vi "SVA 4MV6 T024 CCE.vi"() -> ()   [LabVIEW 2020]
doc: "Ceballos Conde Emanuelm 4MV6 Sistemas de visión artificial 2022/1\nEste vi realiza el control difuso SIMO del sitema de orientacion de un robot lego untilizando el REPERTORIO DE FUNCIONES DEL TOOL KIT FUZZY LOGIC DE LABVIEW."
uses:
  <vilib>/addons/Fuzzy Logic/TypeDefs/FL Defuzzification.ctl
  <vilib>/addons/Fuzzy Logic/TypeDefs/FL Antecedent Connective.ctl
  <vilib>/addons/Fuzzy Logic/TypeDefs/FL Consequent Implication.ctl
  <vilib>/addons/Fuzzy Logic/TypeDefs/FL Modifier.ctl
  <vilib>/addons/Fuzzy Logic/Membership/FL Create Membership Function (Triangle).vi
  <vilib>/addons/Fuzzy Logic/Membership/FL Create Membership Function (Trapezoid).vi
  <vilib>/addons/Fuzzy Logic/FL Fuzzy Controller (SIMO).vi
  <vilib>/addons/Fuzzy Logic/NI_Fuzzy_Logic_API.lvlib
panel:
  out "output values":dbl[](array[numeric])
  out "distancia":dbl(slide) scale=0.0..100.0
  out "angulo":dbl(knob) scale=-25.0..25.0
  in  "Reset":bool
  out "Motor Izquierda":dbl(slide) scale=-100.0..100.0
  out "Motor Derecha":dbl(slide) scale=-100.0..100.0
  out "Plano de trabajo":picture
  in  "stop":bool
  # "Ceballos Conde Emanuel\n4MV6\nSistemas de visión artificial\n2022/1"
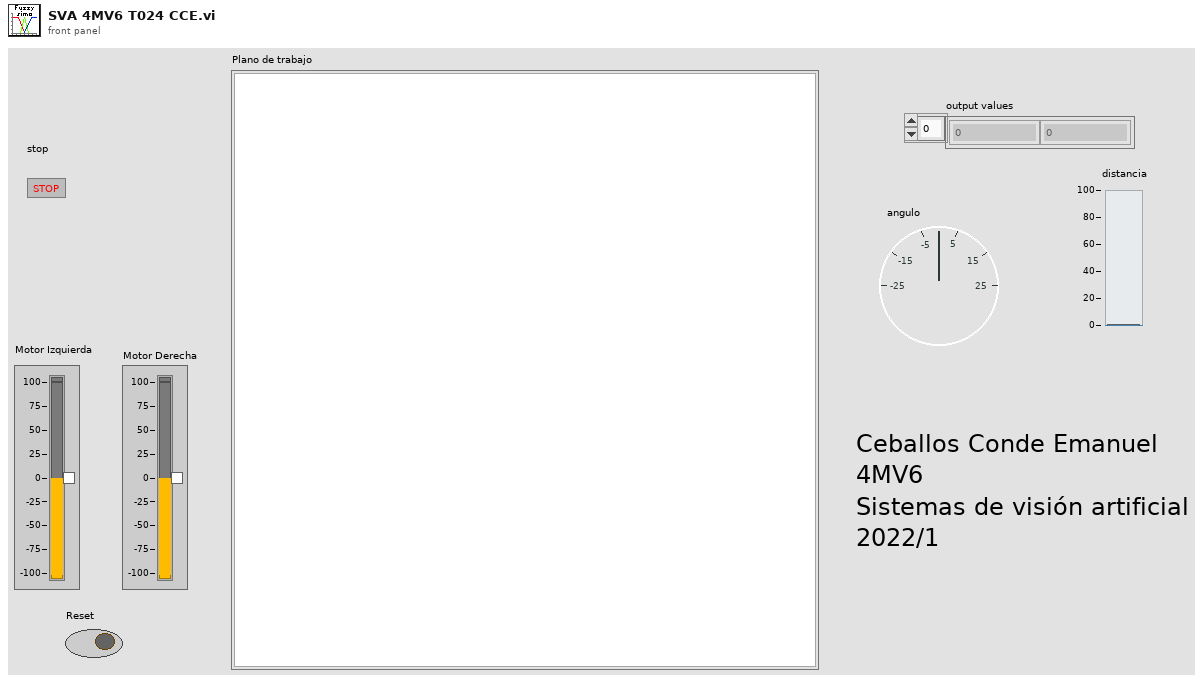
[diagram p1: front panel]
types:
  T1 = typedef "NI_Fuzzy_Logic_API.lvlib/FL Defuzzification.ctl" = u16
  T2 = typedef "NI_Fuzzy_Logic_API.lvlib/FL Membership Function.ctl" = cluster{"name":string, "shape":T3, "points":dbl[], "color":u32, "user-defined shape index":i32}
  T3 = typedef "NI_Fuzzy_Logic_API.lvlib/FL Membership Function Shape.ctl" = u16
  T4 = typedef "NI_Fuzzy_Logic_API.lvlib/FL Variable.ctl" = cluster{"name":string, "range":dbl[], "MFs":T2[]}
  T5 = typedef "NI_Fuzzy_Logic_API.lvlib/FL Modifier.ctl" = u16
  T6 = typedef "NI_Fuzzy_Logic_API.lvlib/FL Consequent Implication.ctl" = u16
  T7 = typedef "NI_Fuzzy_Logic_API.lvlib/FL Antecedent Connective.ctl" = u16
  T8 = typedef "NI_Fuzzy_Logic_API.lvlib/FL Consequent.ctl" = cluster{"Var Index":i32, "MF Index":i32, "Cond":T5}
  T9 = typedef "NI_Fuzzy_Logic_API.lvlib/FL Antecedent.ctl" = cluster{"Var Index":i32, "MF Index":i32, "Cond":T5}
  T10 = typedef "NI_Fuzzy_Logic_API.lvlib/FL Rule.ctl" = cluster{"antecedents":T9[], "antecedent connective":T7, "consequents":T8[], "consequent implication":T6, "degree of support":dbl}
  T11 = typedef "NI_Fuzzy_Logic_API.lvlib/FL System.ctl" = cluster{"input variables":T4[], "output variables":T4[], "rules":T10[], "defuzzification method":T1, "description":string, "user MF interpolating polynomials":T12[]}
  T12 = typedef "NI_Fuzzy_Logic_API.lvlib/FL Interpolating polynomials.ctl" = cluster{"X":dbl[], "Y":dbl[], "Y(x) coeff":dbl[][], "X(y) coeff":dbl[][], "Area(y) coeff":dbl[][], "coa_x(y) coeff":dbl[][]}
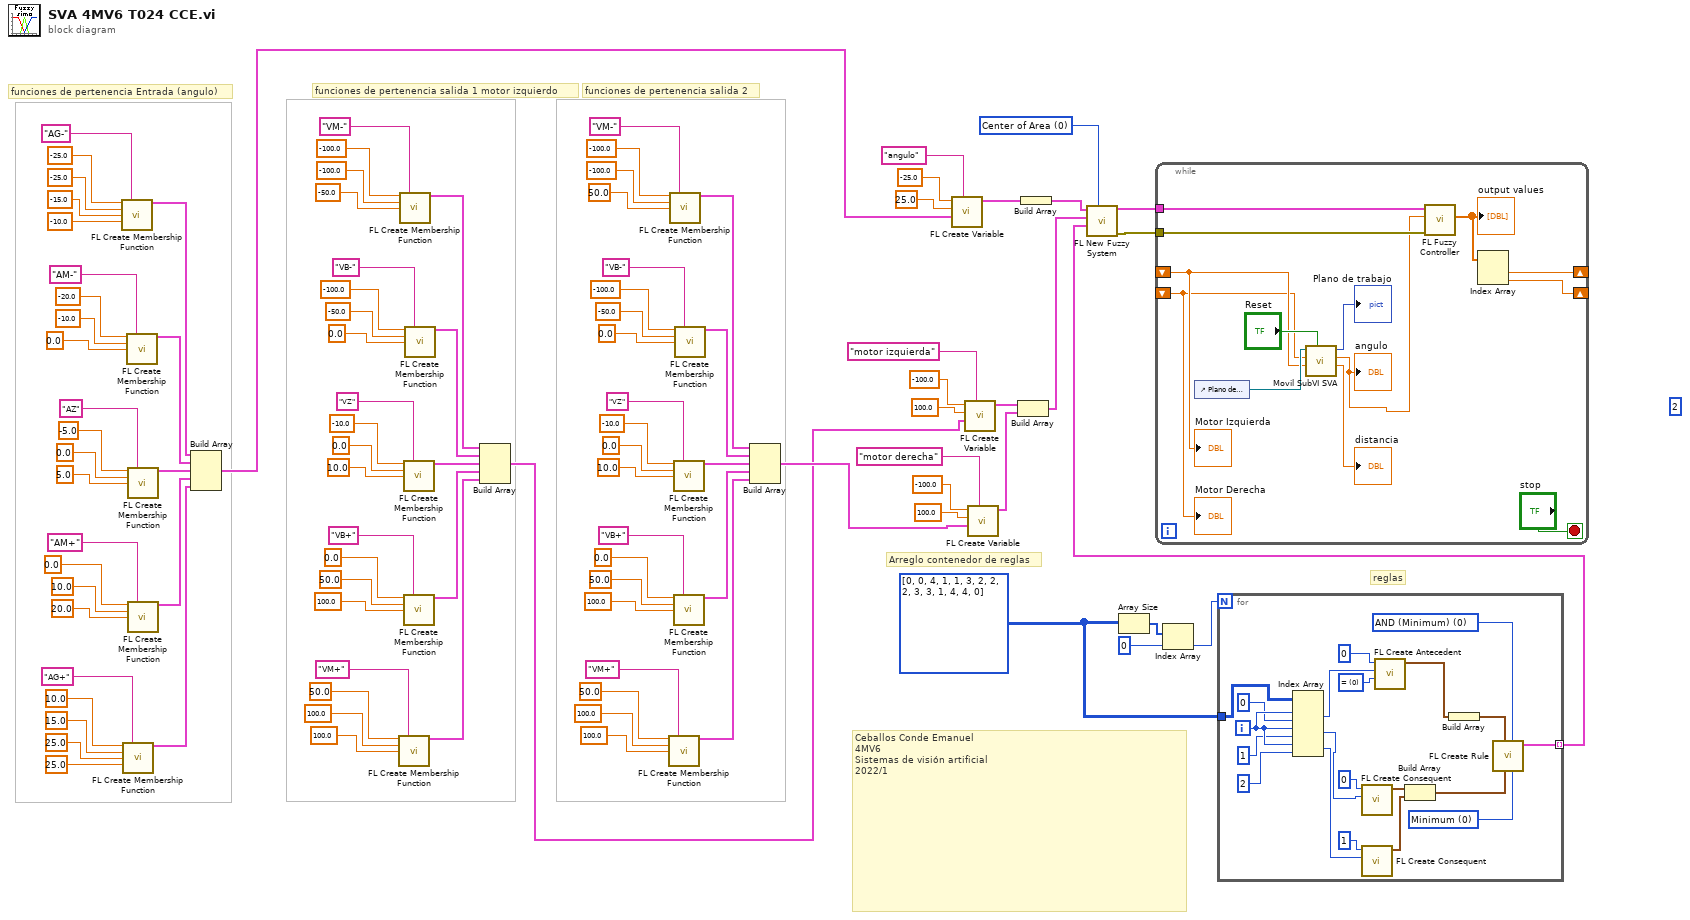
[diagram p0: block diagram]
diagram:
  (unwired) 2
  w4 = i32[][] [[0, 0, 4], [1, 1, 3], [2, 2, 2], [3, 3, 1], [4, 4, 0]]
  w100 = T1 0 items=["Center of Area", "Modified Center of Area", "Center of Sums", "Center of Maximum", "Mean of Maximum"] ("defuzzification method")
  # "Ceballos Conde Emanuel\n4MV6\nSistemas de visión artificial\n2022/1"
  # "Arreglo contenedor de reglas"
  # "funciones de pertenencia salida 2"
  # "funciones de pertenencia salida 1 motor izquierdo"
  # "funciones de pertenencia Entrada (angulo)"
  # "reglas"
  n1 = call-poly <vilib>:"FL Create Membership Function.vi"("left base"=-25.0, "name"="AG-", "left top"=-25.0 ("top"), "right top"=-15.0 ("right base"), "right base"=-10.0) -> ("membership function"=w80:T2)  [unwired: 9 in, 1 out]
  n2 = call-poly <vilib>:"FL Create Membership Function.vi"("left base"=10.0, "name"="AG+", "left top"=15.0 ("top"), "right top"=25.0 ("right base"), "right base"=25.0) -> ("membership function"=w60:T2)  [unwired: 9 in, 1 out]
  n3 = call-poly <vilib>:"FL Create Membership Function.vi"("left base"=-20.0, "name"="AM-", "top"=-10.0, "right base"=0.0) -> ("membership function"=w75:T2)  [unwired: 10 in, 1 out]
  n4 = call-poly <vilib>:"FL Create Membership Function.vi"("left base"=-5.0, "name"="AZ", "top"=0.0, "right base"=5.0) -> ("membership function"=w70:T2)  [unwired: 10 in, 1 out]
  n5 = call-poly <vilib>:"FL Create Membership Function.vi"("left base"=0.0, "name"="AM+", "top"=10.0, "right base"=20.0) -> ("membership function"=w65:T2)  [unwired: 10 in, 1 out]
  n6 = Build Array(w80, w75, w70, w65, w60) -> (w57:T2[])
  n7 = call-poly <vilib>:"FL Create Membership Function.vi"("left base"=50.0, "name"="VM+", "top"=100.0, "right base"=100.0) -> ("membership function"=w32:T2)  [unwired: 10 in, 1 out]
  n8 = call-poly <vilib>:"FL Create Membership Function.vi"("left base"=-100.0, "name"="VM-", "top"=-100.0, "right base"=-50.0) -> ("membership function"=w52:T2)  [unwired: 10 in, 1 out]
  n9 = call-poly <vilib>:"FL Create Membership Function.vi"("left base"=-10.0, "name"="VZ", "top"=0.0, "right base"=10.0) -> ("membership function"=w42:T2)  [unwired: 10 in, 1 out]
  n10 = call-poly <vilib>:"FL Create Membership Function.vi"("left base"=0.0, "name"="VB+", "top"=50.0, "right base"=100.0) -> ("membership function"=w37:T2)  [unwired: 10 in, 1 out]
  n11 = call-poly <vilib>:"FL Create Membership Function.vi"("left base"=-100.0, "name"="VB-", "top"=-50.0, "right base"=0.0) -> ("membership function"=w47:T2)  [unwired: 10 in, 1 out]
  n12 = Build Array(w52, w47, w42, w37, w32) -> (w5:T2[])
  n13 = call-poly <vilib>:"FL Create Membership Function.vi"("left base"=50.0, "name"="VM+", "top"=100.0, "right base"=100.0) -> ("membership function"=w7:T2)  [unwired: 10 in, 1 out]
  n14 = call-poly <vilib>:"FL Create Membership Function.vi"("left base"=-100.0, "name"="VM-", "top"=-100.0, "right base"=50.0) -> ("membership function"=w27:T2)  [unwired: 10 in, 1 out]
  n15 = call-poly <vilib>:"FL Create Membership Function.vi"("left base"=-10.0, "name"="VZ", "top"=0.0, "right base"=10.0) -> ("membership function"=w17:T2)  [unwired: 10 in, 1 out]
  n16 = call-poly <vilib>:"FL Create Membership Function.vi"("left base"=0.0, "name"="VB+", "top"=50.0, "right base"=100.0) -> ("membership function"=w12:T2)  [unwired: 10 in, 1 out]
  n17 = call-poly <vilib>:"FL Create Membership Function.vi"("left base"=-100.0, "name"="VB-", "top"=-50.0, "right base"=0.0) -> ("membership function"=w22:T2)  [unwired: 10 in, 1 out]
  n18 = Build Array(w27, w22, w17, w12, w7) -> (w6:T2[])
  n19 = call <vilib>:"FL Create Variable.vi"("name"="angulo", "membership functions"=w57, "maximum"=25.0, "minimum"=-25.0) -> ("variable"=w96:T4)  [unwired: 6 in, 1 out]
  n20 = call <vilib>:"FL Create Variable.vi"("name"="motor izquierda", "membership functions"=w5, "maximum"=100.0, "minimum"=-100.0) -> ("variable"=w92:T4)  [unwired: 6 in, 1 out]
  n21 = call <vilib>:"FL Create Variable.vi"("name"="motor derecha", "membership functions"=w6, "maximum"=100.0, "minimum"=-100.0) -> ("variable"=w87:T4)  [unwired: 6 in, 1 out]
  n22 = Build Array(w92, w87) -> (w85:T4[])
  n23 = Build Array(w96) -> (w86:T4[])
  n24 = Array Size(array=w4) -> (size(s)=w3:i32[])
  n25 = Index Array(array=w3, index=0) -> (element=w2:i32)
  n26 = for {
    N: w2 -> [_]
    tunnel: [w113] -> w91 mode=indexing
    tunnel: w4 -> [w105]
    i -> [w110]
    w118 = T5 0 items=["=", "!="] ("condition")
    w121 = T6 0 items=["Minimum", "Product"] ("consequent implication")
    w122 = T7 0 items=["AND (Minimum)", "AND (Product)", "OR (Maximum)", "OR (Probabilistic)"] ("antecedent connective")
    n27 = Index Array(array=w105, index (row) #1=w110, index (col) #1=0 ("disabled index (col)"), index (row) #2=w110, index (col) #2=1 ("disabled index (col)"), index (row) #3=w110, index (col) #3=2 ("disabled index (col)")) -> (element #1=w106:i32, element #2=w103:i32, element #3=w104:i32)
    n28 = call <vilib>:"FL Create Consequent.vi"("membership function index"=w103, "variable index"=0) -> ("consequent"=w119:T8)  [unwired: 8 in, 1 out]
    n29 = call <vilib>:"FL Create Consequent.vi"("membership function index"=w104, "variable index"=1) -> ("consequent"=w111:T8)  [unwired: 8 in, 1 out]
    n30 = call <vilib>:"FL Create Antecedent.vi"("condition"=w118, "membership function index"=w106, "variable index"=0) -> ("antecedent"=w120:T9)  [unwired: 7 in, 1 out]
    n31 = Build Array(w119, w111) -> (w114:T8[])
    n32 = Build Array(w120) -> (w115:T9[])
    n33 = call <vilib>:"FL Create Rule.vi"("consequent implication"=w121, "antecedent connective"=w122, "consequents"=w114, "antecedents"=w115) -> ("rule"=w113:T10)  [unwired: 6 in, 1 out]
  }
  n34 = call <vilib>:"FL New Fuzzy System.vi"("defuzzification method"=w100, "rules"=w91, "output variables"=w85, "input variables"=w86) -> ("error out"=w101:errorcluster, "fuzzy system out"=w102:T11)  [unwired: 6 in]
  n35 = while {
    tunnel: w102 -> [w131]
    tunnel: w101 -> [w130]
    shift-right: [w128] -> _
    shift-left: _ -> [w126]
    shift-right: [w127] -> _
    shift-left: _ -> [w125]
    stop <- "stop" stop-if-true
    n36 = control-ref of="Plano de trabajo"() -> (w133:refnum<vi>)
    n37 = call "Movil SubVI SVA.vi"("Reset"="Reset", "Motor Izquierda"=w126, "Motor Derecha"=w125, "Ref Plano"=w133) -> ("Distancia"=→"distancia":dbl, "Angulo"=w123:dbl, "Plano de trabajo"=→"Plano de trabajo":picture)  [unwired: 3 in, 2 out]
    "angulo" <- w123
    n38 = call-poly <vilib>:"FL Fuzzy Controller.vi"("error in (no error)"=w130, "input value"=w123, "fuzzy system in"=w131) -> ("output values"=w129:dbl[])  [unwired: 4 in, 4 out]
    "output values" <- w129
    n39 = Index Array(array=w129) -> (element #1=w128:dbl, element #2=w127:dbl)  [unwired: 2 in]
    "Motor Derecha" <- w125
    "Motor Izquierda" <- w126
  }
